vi "Dialog_Configure Slow Z.vi"(9 "Index of Slow.Z":i32, 10 "Tbl Refnum":refnum<vi>, 11 "Tree Refnum":refnum<vi>) -> (1 "Empty Slow.Z?":bool, 2 "Index of 2DFrame.Scan":i32, 3 "Updated Macro String Array":string[](array[string]))   [LabVIEW 2012]
doc: "SciScan 1.2 160622"
uses:
  FGV_MacroCore_Commands.ctl
  Create Preset commands ENUM.ctl
  GFG/GFGnumericGet.vi
  GFG/GFG library.lvlib
panel:
  in  "OK Button":bool
  out "error out":errorcluster
  in  "error in (no error)":errorcluster
  # "You have selected the Slow.Z Preset. \nThe Macro for carrying out the slow Z-Scan will be auto-generated for you\nbased on the Z-Stack settings  in the main SciScan Interface"
  # "If you need to modify the parameters, select 'Edit' from the Macro GUI\nafter making the necessary changes to Z-Stack parameters\nfrom the SciScan Interface"
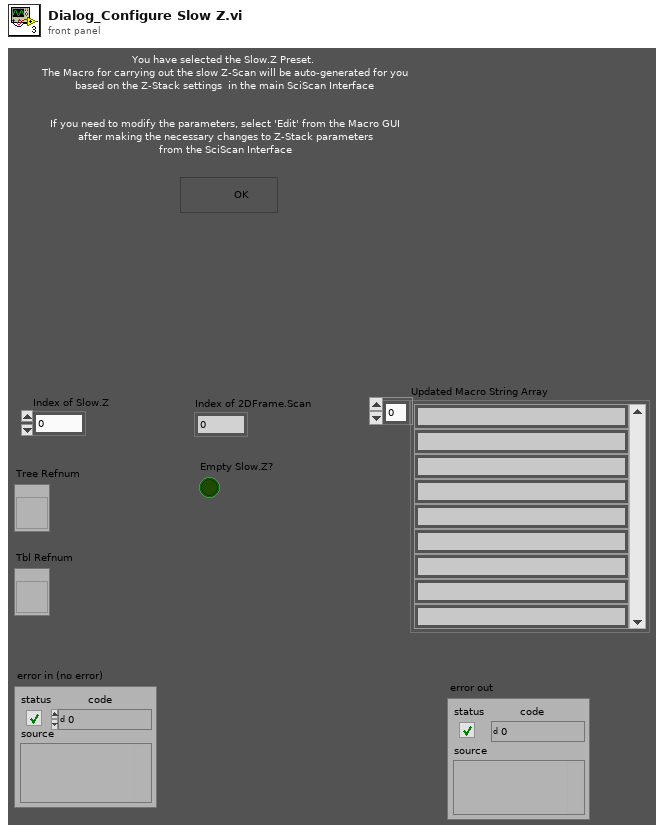
[diagram p1: front panel]
types:
  T1 = typedef "FGV_MacroCore_Commands.ctl" = enum16{"Initialize", "Get Array", "Load macro from file", "Insert Item", "Insert at End", "Edit Parameter String", "Delete instruction", "Move Items", "Save", "SaveAs", "UpdateInfoTable", "Edit Settings File", "New Macro", "Read Temp File", "Delete Multiple"}
  T2 = typedef "Create Preset commands ENUM.ctl" = enum16{"Slow.Z_Move.To.Pos", "Slow.Z_Laser.Power", "Slow.Z_Record", "Tiling_Move.To.Pos", "Tiling_Laser.Power", "Tiling_Record"}
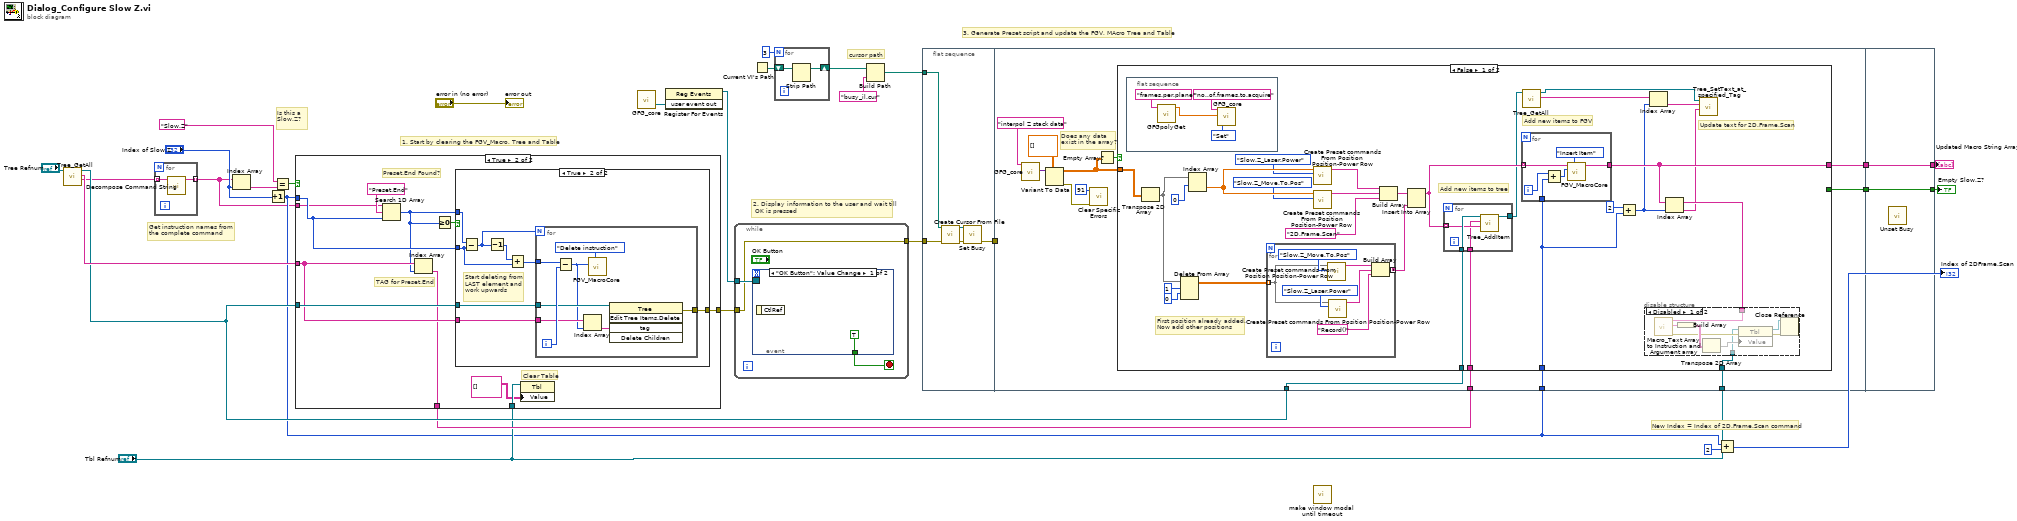
[diagram p0: block diagram]
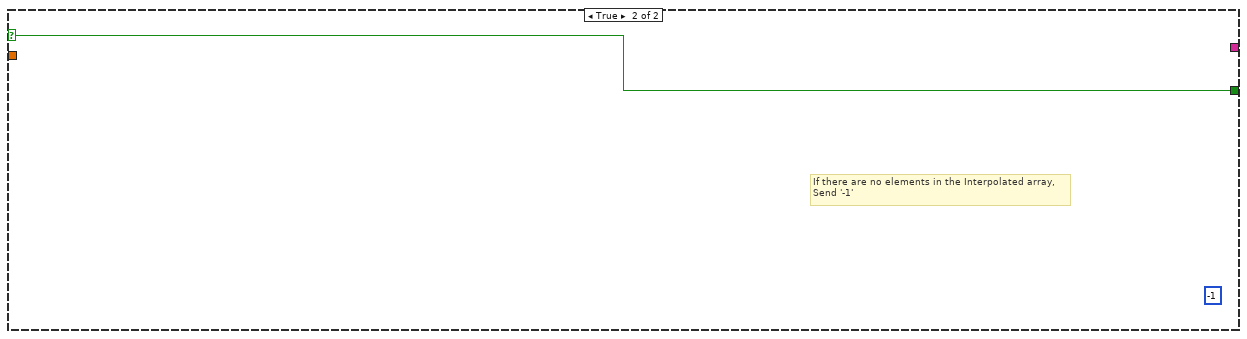
[diagram p3: hidden frame]
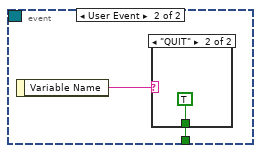
[diagram p6: hidden frame]
diagram:
  # "cursor path"
  # "Get instruction names from\nthe complete command"
  # "New Index = Index of 2D.Frame.Scan command"
  # "3. Generate Preset script and update the FGV, MAcro Tree and Table"
  # "2. Display information to the user and wait till\n OK is pressed"
  # "1. Start by clearing the FGV_Macro, Tree and Table"
  # "Is this a Slow.Z?"
  n1 = call "Tree_GetAll.vi"("Tree Refnum IN"="Tree Refnum") -> ("Text"=w10:string[], "Tags"=w23:string[], "Tree Refnum OUT"=w19:refnum<vi>)  [unwired: 7 in, 1 out]
  n2 = for {
    tunnel: w10 -> [w31] mode=indexing
    tunnel: [w30] -> w9 mode=indexing
    n3 = call "Decompose Command String.vi"("Command IN"=w31) -> ("Action"=w30:string)  [unwired: 7 in, 3 out]
  }
  n4 = Index Array(array=w9, index="Index of Slow.Z") -> (element=w26:string)
  n5 = Increment(x="Index of Slow.Z") -> (x+1=w12:i32)
  n6 = Equal?(x="Slow.Z" ("Variable Name in"), y=w26) -> (x = y?=w24:bool)
  n7 = case shown="True" w24 {
    tunnel: w23 -> [_ w39]
    tunnel: w9 -> [_ w32]
    tunnel: w12 -> [_ w37]
    tunnel: w19 -> [_ w41]
    tunnel: [_ w40] -> w21
    tunnel: [_ w36] -> w18
    tunnel: "Tbl Refnum" -> [_ w34]
    frame False {
    }
    frame True {
      # "Clear Table"
      # "TAG for Preset.End"
      # "Preset.End Found?"
      n8 = Search 1D Array(1D array=w32, element="Preset.End", start index (0)=w37) -> (index of element=w35:i32)
      n9 = Index Array(array=w39, index=w35) -> (element=w36:string)
      n10 = Greater Or Equal To 0?(x=w35) -> (x >= 0?=w38:bool)
      n11 = case shown="True" w38 {
        tunnel: w35 -> [_ w50]
        tunnel: w41 -> [_ w46]
        tunnel: [_ w45] -> w40
        tunnel: w37 -> [_ w44]
        tunnel: w39 -> [_ w43]
        frame False {
        }
        frame True {
          # "Start deleting from LAST element and work upwards"
          n12 = Subtract(x=w50, y=w44) -> (x-y=w49:i32)
          n13 = Decrement(x=w49) -> (x-1=w48:i32)
          n14 = Add(x=w48, y=w44) -> (x+y=w47:i32)
          n15 = for {
            N: w49 -> [_]
            tunnel: w47 -> [w56]
            tunnel: w46 -> [w55]
            tunnel: w43 -> [w54]
            tunnel: [w51] -> w45
            i -> [w57]
            n16 = Subtract(x=w56, y=w57) -> (x-y=w53:i32)
            n17 = Index Array(array=w54, index=w53) -> (element=w52:string)
            n18 = call "FGV_MacroCore.vi"("MacroFGV_Commands"=FGV_MacroCore_Commands."Delete instruction", "Start Index"=w53) -> ()  [unwired: 5 in, 5 out]
            n19 = invoke class="Tree" method="Edit Tree Items.Delete"(reference=w55, "tag"=w52) -> (error out=w51:errorcluster)  [unwired: 3 in, 4 out]
          }
        }
      }
      n20 = property class="Tbl"(reference=w34, "Value"=string[][] []) -> ()  [unwired: 1 in, 2 out]
    }
  }
  n21 = call "GFG_core.vi"() -> ("user event out"=w29:refnum<user-event>)  [unwired: 13 in, 6 out]
  n22 = register-events(w29) -> (reference out=w28:refnum<event-registration>)  [unwired: 2 in, 1 out]
  n23 = while {
    tunnel: w28 -> [w61]
    tunnel: w21 -> [w59]
    tunnel: [w59] -> w20
    stop <- w60 stop-if-true
    n24 = event shown="[0] \"OK Button\": Value Change" {
      selector: w61 -> [_ _]
      dyn-events: _ -> [_ _]
      timeout: _ -> [_ _]
      tunnel: [TRUE w63] -> w60
      event "OK Button": Value Change {
        n25 = event-data() -> ()  [unwired: 1 in, 1 out]
      }
      event User Event {
        n26 = event-data() -> ("Variable Name"=w64:string)  [unwired: 1 in]
        n27 = case shown="\"QUIT\"" w64 {
          tunnel: [_ TRUE] -> w63
          frame "False", Default {
          }
          frame "QUIT" {
          }
        }
      }
    }
  }
  n28 = Current VI's Path() -> (path=w6:path)
  n29 = for {
    N: 3 -> [_]
    shift-right: [w66] -> w5
    shift-left: w6 -> [w67]
    n30 = Strip Path(path=w67) -> (stripped path=w66:path)  [unwired: 1 out]
  }
  n31 = Build Path(base path=w5, name or relative path="busy_il.cur") -> (appended path=w2:path)
  n32 = flat-sequence {
    tunnel: w20 -> [w70]
    tunnel: w2 -> [w69]
    tunnel: [w68] -> w1
    tunnel: w19 -> [w80]
    tunnel: w18 -> [w79]
    tunnel: w12 -> [w78]
    tunnel: "Tbl Refnum" -> [w77]
    tunnel: [w76] -> w8
    tunnel: [w75] -> w7
    tunnel: w1 -> [_]
    tunnel: [w143] -> w14
    tunnel: [w144] -> w15
    tunnel: w8 -> [w144]
    tunnel: w7 -> [w143]
    frame #0 {
      n33 = call <vilib>:"Create Cursor From File.vi"("error in (no error)"=w70, "cursor file"=w69) -> ("error out"=w71:errorcluster, "cursor ID"=w72:refnum<k1>)  [unwired: 8 in]
      n34 = call <vilib>:"Set Busy.vi"("error in (no error)"=w71, "cursor ID"=w72) -> ("error out"=w68:errorcluster)  [unwired: 8 in, 1 out]
    }
    frame #1 {
      # "Does any data exist in the array?"
      n35 = call "GFG_core.vi"("Variable Name in"="interpol Z stack data") -> ("Variant Out"=w85:variant)  [unwired: 12 in, 6 out]
      n36 = Variant To Data(type=dbl[][] [] ("Interpolated Data"), Variant=w85) -> (data=w73:dbl[][], error out=w82:errorcluster)  [unwired: 1 in]
      n37 = call "Clear Specific Errors.vi"("Error In"=w82, "Error number In"=91) -> ()  [unwired: 8 in, 2 out]
      n38 = Empty Array?(array=w73) -> (empty?=w74:bool)
      n39 = case shown="False" w74 {
        selector: w74 -> [_ w142]
        tunnel: w73 -> [w112 _]
        tunnel: w80 -> [w95 _]
        tunnel: w79 -> [w100 _]
        tunnel: w78 -> [w93 _]
        tunnel: w77 -> [w98 _]
        tunnel: [w91 _] -> w76
        tunnel: [_ w142] -> w75
        frame False {
          # "Add new items to FGV"
          # "Update text for 2D.Frame.Scan"
          # "Add new items to tree"
          # "First position already added.\nNow add other positions"
          n40 = flat-sequence {
            frame #0 {
              n41 = call-poly "GFGpolyGet.vi"("Variable Name in"="frames.per.plane") -> ("Numeric"=w139:dbl)  [unwired: 8 in, 2 out]
              n42 = call "GFG_core.vi"("Variable Name in"="no..of.frames.to.acquire", "Variant in"=w139, "Action"=enum16{"Init", "Set", "Get", "Clear"}."Set") -> ()  [unwired: 10 in, 7 out]
            }
          }
          n43 = Transpose 2D Array(2D array=w112) -> (transposed array=w105:dbl[][])
          n44 = Delete From Array(array=w105, length=1, index (row)=0) -> (array with subset deleted=w109:dbl[][])  [unwired: 1 in, 1 out]
          n45 = Index Array(array=w105, index (row)=0) -> (element=w103:dbl[])  [unwired: 1 in]
          n46 = for {
            tunnel: w109 -> [w133] mode=indexing
            tunnel: [w136] -> w106 mode=concatenating
            n47 = call "Create Preset commands From Position Position-Power Row.vi"("Create SlowZ commands_Enum"=Create_Preset_commands_ENUM."Slow.Z_Move.To.Pos", "Position-Power Row"=w133) -> ("concatenated string"=w132:string)  [unwired: 9 in]
            n48 = call "Create Preset commands From Position Position-Power Row.vi"("Create SlowZ commands_Enum"=Create_Preset_commands_ENUM."Slow.Z_Laser.Power", "Position-Power Row"=w133) -> ("concatenated string"=w131:string)  [unwired: 9 in]
            n49 = Build Array(w132, w131, "Record()" ("Variable Name in")) -> (w136:string[])
          }
          n50 = call "Create Preset commands From Position Position-Power Row.vi"("Create SlowZ commands_Enum"=Create_Preset_commands_ENUM."Slow.Z_Laser.Power", "Position-Power Row"=w103) -> ("concatenated string"=w96:string)  [unwired: 9 in]
          n51 = call "Create Preset commands From Position Position-Power Row.vi"("Create SlowZ commands_Enum"=Create_Preset_commands_ENUM."Slow.Z_Move.To.Pos", "Position-Power Row"=w103) -> ("concatenated string"=w97:string)  [unwired: 9 in]
          n52 = Build Array(w96, w97, "2D.Frame.Scan" ("Variable Name in")) -> (w107:string[])
          n53 = Insert Into Array(array=w107, new element=w106) -> (w99:string[])  [unwired: 1 in]
          n54 = for {
            tunnel: w99 -> [w129] mode=indexing
            tunnel: w95 -> [w130]
            tunnel: w100 -> [w128]
            tunnel: [w127] -> w94
            n55 = call "Tree_AddItem.vi"("NEW String"=w129, "Tag at add position"=w128, "Tree Refnum"=w130) -> ("Tree Refnum OUT"=w127:refnum<vi>)  [unwired: 6 in, 2 out]
          }
          n56 = for {
            tunnel: w99 -> [w125] mode=indexing
            tunnel: [w122] -> w91
            tunnel: w93 -> [w123]
            i -> [w124]
            n57 = Add(x=w124, y=w123) -> (x+y=w121:i32)
            n58 = call "FGV_MacroCore.vi"("MacroFGV_Commands"=FGV_MacroCore_Commands."Insert Item", "Start Index"=w121, "Macro Command or Info (String)"=w125) -> ("Macro String Array"=w122:string[])  [unwired: 4 in, 4 out]
          }
          n59 = call "Tree_GetAll.vi"("Tree Refnum IN"=w94) -> ("Tags"=w90:string[], "Tree Refnum OUT"=w87:refnum<vi>)  [unwired: 7 in, 2 out]
          n60 = Add(x=2 ("y"), y=w93) -> (x+y=w89:i32)
          n61 = disable-structure shown="Disabled" {
            disable-tunnel: w98 -> [w114 _]
            disable-tunnel: w91 -> [w113 _]
            frame Disabled {
              n62 = call "Macro_Text Array to Instruction and Argument array.vi"("Macro Array IN"=w113) -> ("Error Out"=w116:errorcluster, "Argument List (Txt)"=w115:string[])  [unwired: 8 in, 1 out]
              n63 = Build Array(w115) -> (w118:string[][])
              n64 = Transpose 2D Array(2D array=w118) -> (transposed array=w117:string[][])
              n65 = property class="Tbl"(reference=w114, error in=w116, "Value"=w117) -> (reference out=w119:refnum<vi>, error out=w120:errorcluster)
              n66 = Close Reference(reference=w119, error in (no error)=w120) -> ()  [unwired: 1 out]
            }
            frame Enabled {
            }
          }
          n67 = Index Array(array=w90, index=w89) -> (element=w88:string)
          n68 = Index Array(array=w91, index=w89) -> (element=w86:string)
          n69 = call "Tree_SetText_at_specified_Tag.vi"("New String IN"=w86, "Tag (whose string to be edited)"=w88, "Tree Refnum IN"=w87) -> ()  [unwired: 7 in, 2 out]
        }
        frame True {
          (unwired) -1
          # "If there are no elements in the Interpolated array,\nSend '-1'"
        }
      }
    }
    frame #2 {
      n70 = call <vilib>:"Unset Busy.vi"() -> ()  [unwired: 11 in, 1 out]
    }
  }
  n71 = call "make window modal until timeout.vi"() -> ()  [unwired: 12 in]
  n72 = Add(x=w12, y=2) -> (x+y=→"Index of 2DFrame.Scan":i32)
  "error out" <- "error in (no error)"
  "Updated Macro String Array" <- w15
  "Empty Slow.Z?" <- w14
